vi "Find Unique SensorIDs.vi"(8 "error in (no error)":errorcluster, 11 "Calibration Points in":T1[](array[typedef])) -> (0 "error out":errorcluster, 3 "SensorIDs":i32[](array[numeric]))   [LabVIEW 2026, in "Analysis.lvlib"]
uses:
  controls/Messaging Payloads/Calibration Point Table Insert.ctl
  Analysis.lvlib
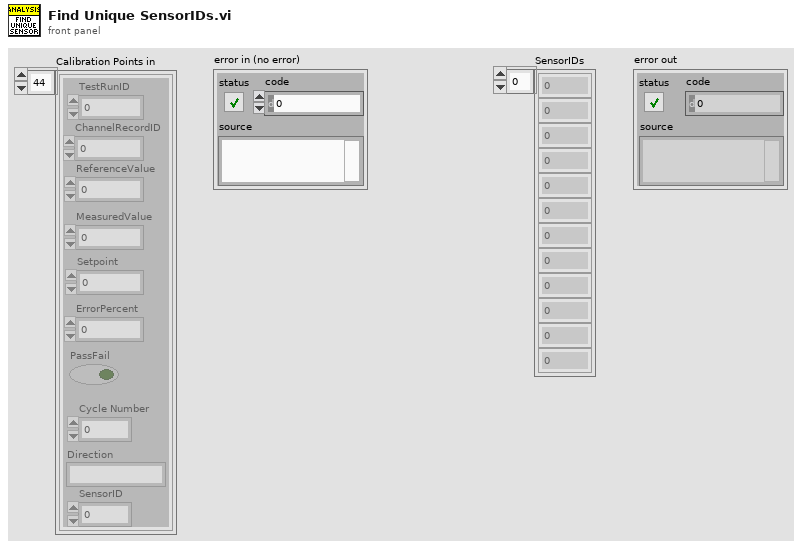
[diagram p1: front panel]
types:
  T1 = typedef "Calibration Point Table Insert.ctl" = cluster{"TestRunID":i32, "ChannelRecordID":i32, "Setpoint":dbl, "MeasuredValue":dbl, "ErrorPercent":dbl, "PassFail":bool, "ReferenceValue":dbl, "Cycle Number":i32, "Direction":string, "SensorID":i32}
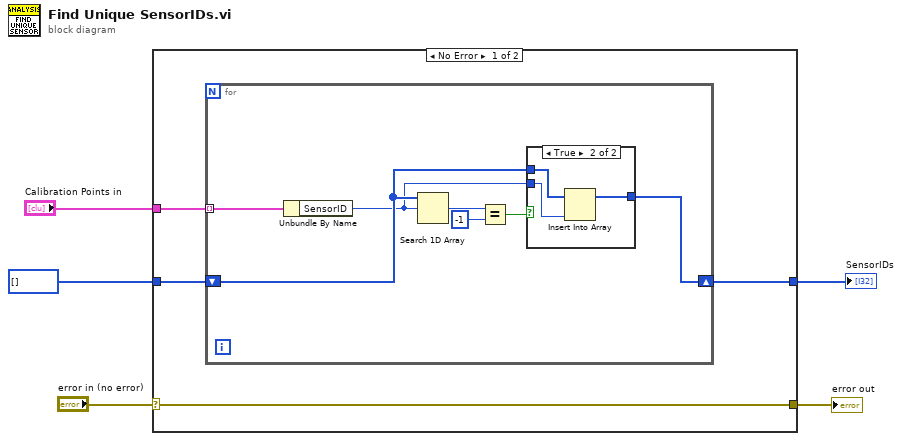
[diagram p0: block diagram]
diagram:
  n1 = case shown="No Error" "error in (no error)" {
    selector: "error in (no error)" -> [w6 w21]
    tunnel: "Calibration Points in" -> [w9 _]
    tunnel: i32[] [] -> [w8 w22]
    tunnel: [w7 w22] -> w4
    tunnel: [w6 w21] -> w2
    frame No Error {
      n2 = for {
        tunnel: w9 -> [w16] mode=indexing
        shift-right: [w15] -> w7
        shift-left: w8 -> [w14]
        n3 = Unbundle By Name(w16) -> ("SensorID"=w10:i32)
        n4 = Search 1D Array(1D array=w14, element=w10) -> (index of element=w13:i32)  [unwired: 1 in]
        n5 = Equal?(x=w13, y=-1) -> (x = y?=w11:bool)
        n6 = case shown="True" w11 {
          tunnel: [w17 w20] -> w15
          tunnel: w14 -> [w17 w19]
          tunnel: w10 -> [_ w18]
          frame False {
          }
          frame True {
            n7 = Insert Into Array(array=w19, new element=w18) -> (w20:i32[])  [unwired: 1 in]
          }
        }
      }
    }
    frame Error {
    }
  }
  "SensorIDs" <- w4
  "error out" <- w2
